vi "S7COMM - Create JOB Message Header.vi"(9 "S7 Data Length":u16, 10 "S7 Parameters Length":u16, 11 "Sequence Number":u16) -> (3 "S7 JOB Header":u8[](array[numeric]))   [LabVIEW 2014, in "S7NetCom.lvclass"]
doc: "S7 Header\n_____\nCopyright (c) 2019 Hampel Software Engineering (HSE), released under BSD license. More info can be found on https://dokuwiki.hampel-soft.com/code/hse/s7netcom. Original code published by Marc Christenson, Sisu Devices."
uses:
  S7NetCom.lvclass
  S7COMM - Message Types--ring.ctl
panel:
  # "More info on https://dokuwiki.hampel-soft.com/code/hse/s7netcom\n\nCopyright (c) 2019, HAMPEL SOFTWARE ENGINEERING (HSE)\nOriginal code developed by Marc Christenson, Sisu Devices\nAll rights reserved.\n\nRedistribution and use in source and binary forms, with or without\nmodification, are permitted provided that the following conditions are met:\n\n1. Redistributions of source code must retain the above copyright\n   notice, this list of conditions and the following disclaimer.\n\n2. Redistributions in binary form must reproduce the above copyright\n   notice, this list of conditions and the following disclaimer in the\n   documentation and/or other materials provided with the distribution.\n\n3. All advertising materials mentioning features or use of this software\n   must display the following acknowledgement:\n   This product includes software developed by HAMPEL SOFTWARE ENGINEERING.\n\n4. Neither the name of HAMPEL SOFTWARE ENGINEERING nor the\n   names of its contributors may be used to endorse or promote products\n   derived from this software without specific prior written permission.\n\nTHIS SOFTWARE IS PROVIDED BY HAMPEL SOFTWARE ENGINEERING ''AS IS'' AND ANY\nEXPRESS OR IMPLIED WARRANTIES, INCLUDING, BUT NOT LIMITED TO, THE IMPLIED\nWARRANTIES OF MERCHANTABILITY AND FITNESS FOR A PARTICULAR PURPOSE ARE\nDISCLAIMED. IN NO EVENT SHALL HAMPEL SOFTWARE ENGINEERING BE LIABLE FOR ANY\nDIRECT, INDIRECT, INCIDENTAL, SPECIAL, EXEMPLARY, OR CONSEQUENTIAL DAMAGES\n(INCLUDING, BUT NOT LIMITED TO, PROCUREMENT OF SUBSTITUTE GOODS OR SERVICES;\nLOSS OF USE, DATA, OR PROFITS; OR BUSINESS INTERRUPTION) HOWEVER CAUSED AND\nON ANY THEORY OF LIABILITY, WHETHER IN CONTRACT, STRICT LIABILITY, OR TORT\n(INCLUDING NEGLIGENCE OR OTHERWISE) ARISING IN ANY WAY OUT OF THE USE OF THIS\nSOFTWARE, EVEN IF ADVISED OF THE POSSIBILITY OF SUCH DAMAGE."
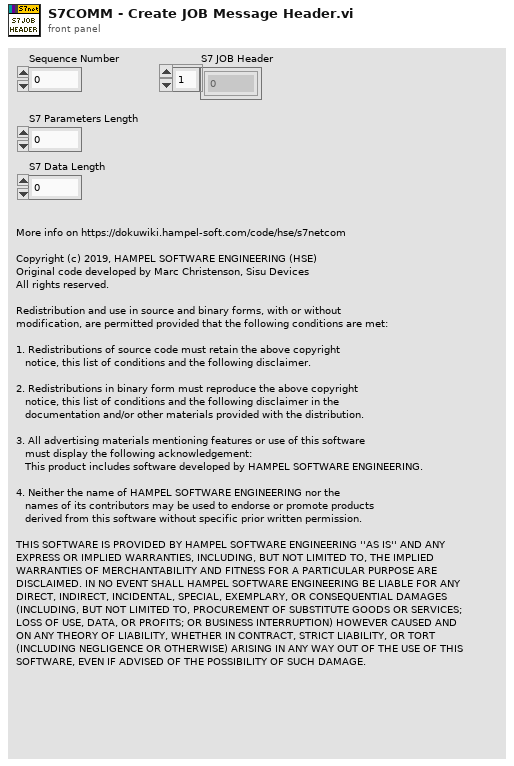
[diagram p1: front panel]
types:
  T1 = typedef "S7NetCom.lvclass/S7COMM - Message Types--ring.ctl" = u8
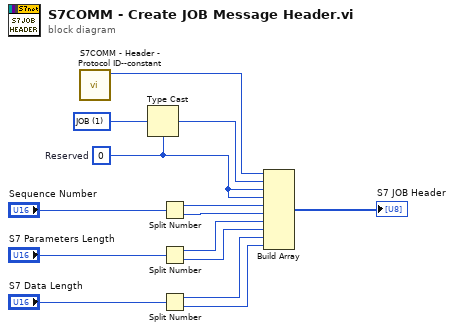
[diagram p0: block diagram]
diagram:
  w1 = u8 0  # Reserved
  w3 = T1 1 items=["JOB"=1, "ACK"=2, "ACK_DATA"=3, "USERDATA"=7] ("Message Type")
  n1 = call "S7COMM - Header - Protocol ID--constant.vi"() -> ("Protocol ID"=w4:u8)  [unwired: 11 in]
  n2 = Type Cast(type=w1, x=w3) -> (*(type *) &x=w2:u8)
  n3 = Split Number(x="Sequence Number") -> (hi(x)=w13:u8, lo(x)=w12:u8)
  n4 = Split Number(x="S7 Parameters Length") -> (hi(x)=w11:u8, lo(x)=w10:u8)
  n5 = Split Number(x="S7 Data Length") -> (hi(x)=w7:u8, lo(x)=w6:u8)
  n6 = Build Array(w4, w2, w1, w1, w13, w12, w11, w10, w7, w6) -> (→"S7 JOB Header":u8[])
